vi "autoBuild.vi"() -> ()   [LabVIEW 2015]
uses:
  <vilib>/AppBuilder/AB_API_Simple/Build (path).vi
  <vilib>/AppBuilder/AB_API_Simple/NI_App_Builder_API.lvlib
panel:
  out "Generated files":path[](array[path])
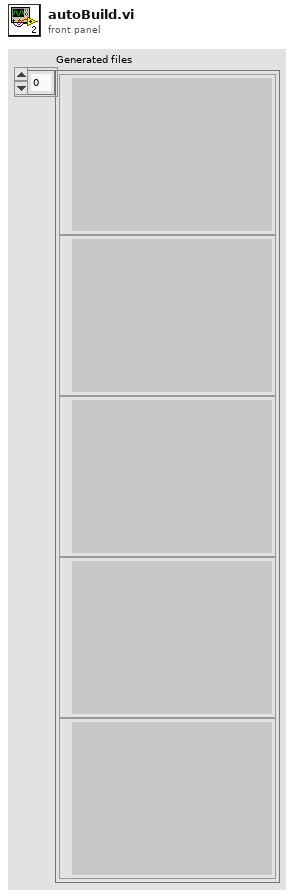
[diagram p1: front panel]
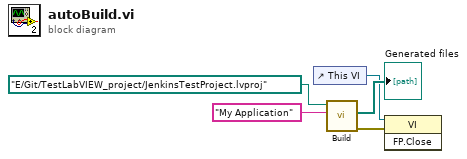
[diagram p0: block diagram]
diagram:
  n1 = control-ref of="This VI"() -> (w2:refnum<vi>)
  n2 = call-poly <vilib>:"Build.vi"("Name of build specification (if empty: build all)"="My Application", "Path to project"=path "E:/Git/TestLabVIEW_project/JenkinsTestProject.lvproj") -> ("error out"=w1:errorcluster, "Generated files"=→"Generated files":path[])  [unwired: 8 in]
  n3 = invoke class="VI" method="FP.Close"(reference=w2, error in=w1) -> ()  [unwired: 1 in, 3 out]
